vi "Input Control.vi"(3 "Device":enum16{"Joysticks", "Controller"}(ring), 5 "State":enum16{"Open", "Run", "End"}(ring)) -> (0 "Joystick 2":T2, 1 "Joystick 1":T2, 2 "Controller":T3)   [LabVIEW 2013]
doc: "This VI will initialize human interface devices for use with the robot. It is compatible with any device provided your PC has the proper drivers installed. It has been specifically written to function with either a gamepad or dual joysticks, but will function with any devices. It can get values for up to 6 axes and 12 buttons per device, and if the devices used are one of the kinds of devices that this VI was specifically written for, you will have the added bonus of prenamed outputs! For two input devices to be controlled simultaniously, use the \"Joysticks\" device input. If you only need one, esp. if the device is a gamepad, use the \"Controller\" device input setting. Two gamepads CAN be operated simultaniously by this VI, but you will not have the niceties of axes pregrouped into their respective joysticks.\n\nThe following inputs are required:\n State must be \"Open\" when initializing, \"Run\" when output values are necessary, and \"End\" at the end of your program.\n Device must be specified as described above.\n\nThe following outputs are required when the Device input is set to \"Joysticks\" to recieve data:\n Joystick 1 must be wired to an \"Unbundle\" block followed by two more \"Unbundle\" blocks to get the individual values. Use \"Unbundle By Name\" to use the names associated with the outputs.\n Joystick 2 must be wired to an \"Unbundle\" block followed by two more \"Unbundle\" blocks to get the individual values. Use \"Unbundle By Name\" to use the names associated with the outputs.\n\nThe following outputs are required when the Device input is set to \"Controller\" to recieve data:\n Controller must be wired to an \"Unbundle\" block followed by another \"Unbundle\" block for each data wire. The \"Axes\" subcluster contains two more clusters which contain the joystick values. \"Unbundle\" them to get values for the joysticks. The triggers (axis 3) are not contained within a subcluster of \"Axes\" and their value is available immediately."
uses:
  <vilib>/Rock Robotics/WPI/Joystick/WPI_JoystickButtonState.ctl
  <vilib>/Rock Robotics/WPI/Joystick/WPI_JoystickDeviceEnum.ctl
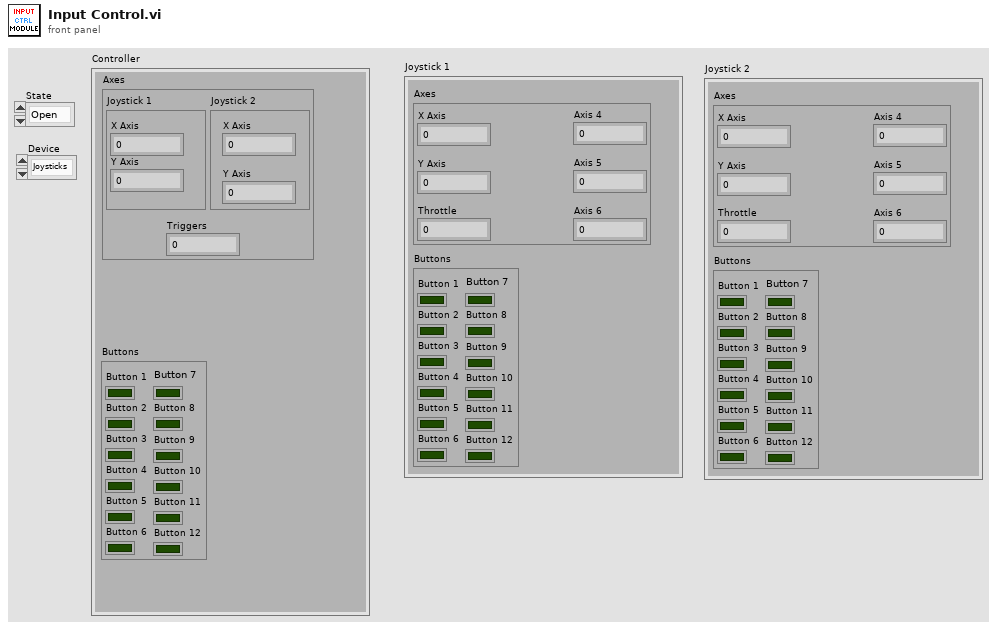
[diagram p1: front panel]
types:
  T1 = typedef "WPI_JoystickButtonState.ctl" = cluster{"Button 1":bool, "Button 2":bool, "Button 3":bool, "Button 4":bool, "Button 5":bool, "Button 6":bool, "Button 7":bool, "Button 8":bool, "Button 9":bool, "Button 10":bool, "Button 11":bool, "Button 12":bool}
  T2 = cluster{"Axes":cluster{"X Axis":dbl, "Y Axis":dbl, "Throttle":dbl, "Axis 4":dbl, "Axis 5":dbl, "Axis 6":dbl}, "Buttons":T1}
  T3 = cluster{"Axes":cluster{"Triggers":dbl, "Joystick 1":cluster{"X Axis":dbl, "Y Axis":dbl}, "Joystick 2":cluster{"X Axis":dbl, "Y Axis":dbl}}, "Buttons":T1}
  T4 = typedef "WPI_JoystickDeviceEnum.ctl" = enum16{"USB 1", "USB 2", "USB 3", "USB 4", "Kinect 1", "Kinect 2"}
  T5 = typedef "WPI_JoystickDevRef.ctl" = cluster{"Device":T4}
  T6 = cluster{"axis 1 (x)":dbl, "axis 2 (y)":dbl, "axis 3 (throttle)":dbl, "axis 4":dbl, "axis 5":dbl, "axis 6":dbl}
  T7 = cluster{"Axes":cluster{"axis 1 (x)":dbl, "axis 2 (y)":dbl, "axis 3 (throttle)":dbl, "axis 4":dbl, "axis 5":dbl, "axis 6":dbl}, "Buttons":T1}
  T8 = cluster{"axis 3 (throttle)":dbl, cluster{"axis 1 (x)":dbl, "axis 2 (y)":dbl}, cluster{"axis 4":dbl, "axis 5":dbl}}
  T9 = cluster{cluster{"axis 3 (throttle)":dbl, cluster{"axis 1 (x)":dbl, "axis 2 (y)":dbl}, cluster{"axis 4":dbl, "axis 5":dbl}}, "Buttons":T1}
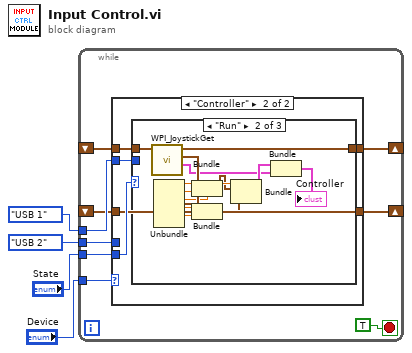
[diagram p0: block diagram]
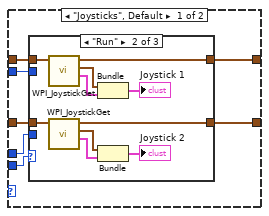
[diagram p2: hidden frame]
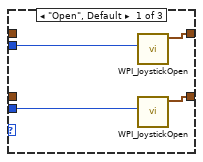
[diagram p3: hidden frame]
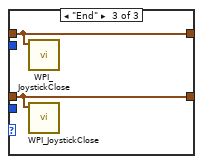
[diagram p4: hidden frame]
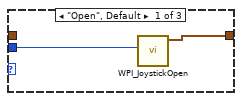
[diagram p5: hidden frame]
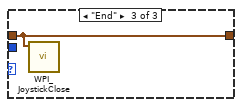
[diagram p6: hidden frame]
diagram:
  n1 = while {
    tunnel: "State" -> [w13]
    shift-right: [w12] -> _
    shift-left: _ -> [w11]
    tunnel: "Device" -> [w9]
    tunnel: WPI_JoystickDeviceEnum."USB 1" ("Controller") -> [w8]
    shift-right: [w7] -> _
    shift-left: _ -> [w6]
    tunnel: WPI_JoystickDeviceEnum."USB 2" ("Controller") -> [w5]
    stop <- TRUE stop-if-true
    n2 = case shown="\"Controller\"" w9 {
      tunnel: w13 -> [w18 w41]
      tunnel: [w16 w40] -> w12
      tunnel: w11 -> [w15 w39]
      tunnel: w8 -> [w17 w38]
      tunnel: [w20 w37] -> w7
      tunnel: w6 -> [w14 w37]
      tunnel: w5 -> [w19 _]
      frame "Joysticks", Default {
        n3 = case shown="\"Run\"" w18 {
          tunnel: [w24 w34 w36] -> w16
          tunnel: [w23 w31 w35] -> w20
          tunnel: w19 -> [w22 _ _]
          tunnel: w17 -> [w21 _ _]
          tunnel: w15 -> [_ w33 w36]
          tunnel: w14 -> [_ w32 w35]
          frame "Open", Default {
            n4 = call <vilib>:"WPI_JoystickOpen.vi"("JoystickDevice"=w21) -> ("JoystickDevRef"=w24:T5)  [unwired: 10 in]
            n5 = call <vilib>:"WPI_JoystickOpen.vi"("JoystickDevice"=w22) -> ("JoystickDevRef"=w23:T5)  [unwired: 10 in]
          }
          frame "Run" {
            n6 = call <vilib>:"WPI_JoystickGet.vi"("JoystickDevRef"=w33) -> ("Buttons"=w30:T1, "Axes"=w29:T6, "JoystickDevRef"=w34:T5)  [unwired: 4 in]
            n7 = call <vilib>:"WPI_JoystickGet.vi"("JoystickDevRef"=w32) -> ("Buttons"=w26:T1, "Axes"=w27:T6, "JoystickDevRef"=w31:T5)  [unwired: 4 in]
            n8 = Bundle("Axes"=w29, "Buttons"=w30) -> (→"Joystick 1":T7)  [unwired: 1 in]
            n9 = Bundle("Axes"=w27, "Buttons"=w26) -> (→"Joystick 2":T7)  [unwired: 1 in]
          }
          frame "End" {
            n10 = call <vilib>:"WPI_JoystickClose.vi"("JoystickDevRef"=w36) -> ()  [unwired: 11 in]
            n11 = call <vilib>:"WPI_JoystickClose.vi"("JoystickDevRef"=w35) -> ()  [unwired: 11 in]
          }
        }
      }
      frame "Controller" {
        n12 = case shown="\"Run\"" w41 {
          tunnel: [w43 w55 w57] -> w40
          tunnel: w39 -> [_ w56 w57]
          tunnel: w38 -> [w42 _ _]
          frame "Open", Default {
            n13 = call <vilib>:"WPI_JoystickOpen.vi"("JoystickDevice"=w42) -> ("JoystickDevRef"=w43:T5)  [unwired: 10 in]
          }
          frame "Run" {
            n14 = call <vilib>:"WPI_JoystickGet.vi"("JoystickDevRef"=w56) -> ("Buttons"=w47:T1, "Axes"=w54:T6, "JoystickDevRef"=w55:T5)  [unwired: 4 in]
            n15 = Unbundle(w54) -> ("axis 1 (x)"=w50:dbl, "axis 2 (y)"=w51:dbl, "axis 3 (throttle)"=w45:dbl, "axis 4"=w53:dbl, "axis 5"=w52:dbl)  [unwired: 1 out]
            n16 = Bundle("axis 1 (x)"=w50, "axis 2 (y)"=w51) -> (w44:cluster{"axis 1 (x)":dbl, "axis 2 (y)":dbl})  [unwired: 1 in]
            n17 = Bundle("axis 4"=w53, "axis 5"=w52) -> (w49:cluster{"axis 4":dbl, "axis 5":dbl})  [unwired: 1 in]
            n18 = Bundle("axis 3 (throttle)"=w45, w44, w49) -> (w48:T8)  [unwired: 1 in]
            n19 = Bundle(w48, "Buttons"=w47) -> (→"Controller":T9)  [unwired: 1 in]
          }
          frame "End" {
            n20 = call <vilib>:"WPI_JoystickClose.vi"("JoystickDevRef"=w57) -> ()  [unwired: 11 in]
          }
        }
      }
    }
  }
